vi "Prepare Paths For Expiration Check.vi"(0 "Scalar SG Path Group in":refnum<class "SG 18GHz Path Group.lvclass">, 5 "TSM Context":T1, 11 "error in (no error)":errorcluster) -> (4 "Scalar SG Path Group out":refnum<class "SG 18GHz Path Group.lvclass">, 15 "error out":errorcluster)   [LabVIEW 2023, in "RFFixtureCharact.RFPM.lvlib" / "SG 18GHz Path Group.lvclass"]
uses:
  SG 18GHz Path Group.lvclass
  C:/srd-semi-rfcal-software/AuxTools/STSRFFixtureCharactUtility/Source/Code Modules/Common/Base Classes/Path Group/Path Group.lvclass
  <vilib>/NI_TestStand_SemiconductorModule/NI_TestStand_Semiconductor_Module.lvlibp/PinMap/General/SemiconductorModuleContext.ctl
  Paths/SG Path/SG 18GHz Path.lvclass
  C:/srd-semi-rfcal-software/AuxTools/STSRFFixtureCharactUtility/Source/Code Modules/Common/Base Classes/Path/Path.lvclass
  Charact Result Accessor/Scalar/Scalar Charact Result Accessor.lvclass
  C:/srd-semi-rfcal-software/AuxTools/STSRFFixtureCharactUtility/Source/Code Modules/Fixture/RFPM/Charact Result Accessor/Base/Charact Result Accessor.lvclass
  C:/srd-semi-rfcal-software/AuxTools/STSRFFixtureCharactUtility/Source/Code Modules/Common/Result Accessor/Result Accessor.lvclass
  <vilib>/NI_TestStand_SemiconductorModule/NI_TestStand_Semiconductor_Module.lvlibp/PinMap/RF/RFSG/PinToNIRFSGSession.vi
  Common/Base Classes/Path/Path.lvclass
  Common/Result Accessor/Result Accessor.lvclass
  <vilib>/NI_TestStand_SemiconductorModule/NI_TestStand_Semiconductor_Module.lvlibp
  Common/Base Classes/Path Group/Path Group.lvclass
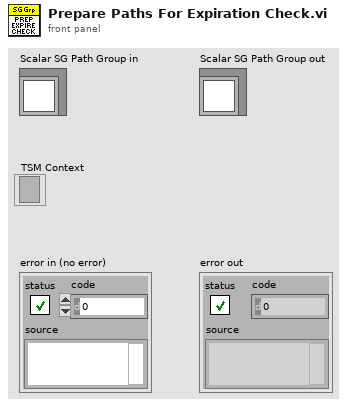
[diagram p1: front panel]
types:
  T1 = typedef "NI_TestStand_Semiconductor_Module.lvlibp/SemiconductorModuleContext.ctl" = refnum<k7>
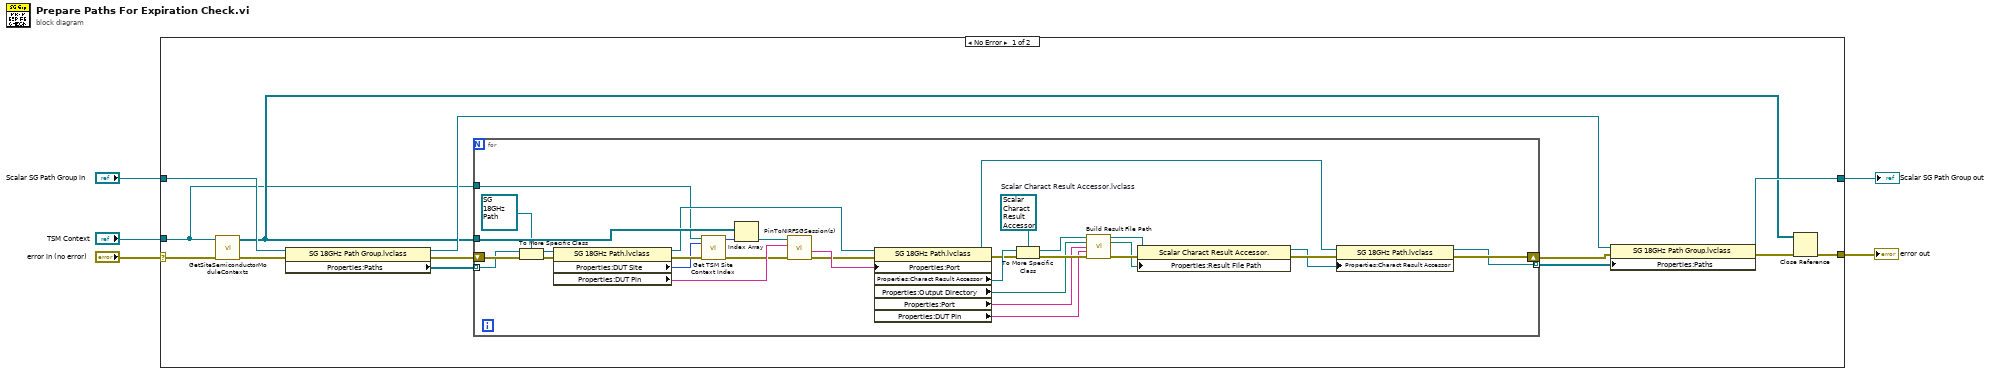
[diagram p0: block diagram]
diagram:
  n1 = case shown="No Error" "error in (no error)" {
    selector: "error in (no error)" -> [w8 w52]
    tunnel: "TSM Context" -> [w7 _]
    tunnel: "Scalar SG Path Group in" -> [w11 w51]
    tunnel: [w10 w52] -> w2
    tunnel: [w12 w51] -> w1
    frame No Error {
      n2 = call <vilib>:"GetSiteSemiconductorModuleContexts.vi"("error in (no error)"=w8, "Semiconductor Module Context"=w7) -> ("error out"=w16:errorcluster, "Site Semiconductor Module Contexts"=w9:T1[])  [unwired: 8 in]
      n3 = property class="SG 18GHz Path Group.lvclass"(reference=w11, error in=w16) -> (reference out=w14:refnum<class "SG 18GHz Path Group.lvclass">, error out=w18:errorcluster, "Properties:Paths"=w17:refnum<class "Path.lvclass">[])
      n4 = for {
        tunnel: w9 -> [w50]
        tunnel: w17 -> [w42] mode=indexing
        tunnel: [w29] -> w13 mode=indexing
        tunnel: w7 -> [w35]
        shift-right: [w30] -> w6
        shift-left: w18 -> [w44]
        w34 = refnum<class "Scalar Charact Result Accessor.lvclass"> refnum  # Scalar Charact Result Accessor.lvclass
        n5 = To More Specific Class(target class=refnum<class "SG 18GHz Path.lvclass"> refnum ("STS Scalar Fixture Characterization.lvlib:Scalar SG Path.lvclass"), reference=w42, error in=w44) -> (specific class reference=w40:refnum<class "SG 18GHz Path.lvclass">, error out=w43:errorcluster)
        n6 = property class="SG 18GHz Path.lvclass"(reference=w40, error in=w43) -> (reference out=w45:refnum<class "SG 18GHz Path.lvclass">, error out=w47:errorcluster, "Properties:DUT Site"=w37:i32, "Properties:DUT Pin"=w39:string)
        n7 = call "Get TSM Site Context Index.vi"("Semiconductor Module Context"=w35, "Site Number"=w37, "error in (no error)"=w47) -> ("index of Site TSM Context"=w36:i32, "error out"=w38:errorcluster)  [unwired: 11 in]
        n8 = Index Array(array=w50, index=w36) -> (element=w48:T1)
        n9 = call-poly <vilib>:"PinToNIRFSGSession(s).vi"("error in (no error)"=w38, "Pin"=w39, "Semiconductor Module Context"=w48) -> ("error out"=w46:errorcluster, "Port"=w49:string)  [unwired: 4 in, 3 out]
        n10 = property class="SG 18GHz Path.lvclass"(reference=w45, error in=w46, "Properties:Port"=w49) -> (reference out=w27:refnum<class "SG 18GHz Path.lvclass">, error out=w28:errorcluster, "Properties:Charact Result Accessor"=w31:refnum<class "Result Accessor.lvclass">, "Properties:Output Directory"=w22:path, "Properties:Port"=w21:string, "Properties:DUT Pin"=w20:string)
        n11 = To More Specific Class(target class=w34, reference=w31, error in=w28) -> (specific class reference=w23:refnum<class "Scalar Charact Result Accessor.lvclass">, error out=w26:errorcluster)
        n12 = call-dynamic "Build Result File Path.vi"("Charact Result Accessor in"=w23, "Output Directory"=w22, "Port 1"=w21, "Port 2"=w20, "error in"=w26) -> ("Charact Result Accessor out"=w19:refnum<class "Scalar Charact Result Accessor.lvclass">, "Result File Path"=w24:path, "error out"=w25:errorcluster)  [unwired: 8 in]
        n13 = property class="Scalar Charact Result Accessor."(reference=w19, error in=w25, "Properties:Result File Path"=w24) -> (reference out=w32:refnum<class "Scalar Charact Result Accessor.lvclass">, error out=w33:errorcluster)
        n14 = property class="SG 18GHz Path.lvclass"(reference=w27, error in=w33, "Properties:Charact Result Accessor"=w32) -> (reference out=w29:refnum<class "SG 18GHz Path.lvclass">, error out=w30:errorcluster)
      }
      n15 = property class="SG 18GHz Path Group.lvclass"(reference=w14, error in=w6, "Properties:Paths"=w13) -> (reference out=w12:refnum<class "SG 18GHz Path Group.lvclass">, error out=w15:errorcluster)
      n16 = Close Reference(reference=w9, error in (no error)=w15) -> (error out=w10:errorcluster)
    }
    frame Error {
    }
  }
  "error out" <- w2
  "Scalar SG Path Group out" <- w1
